vi "NI 9234 Calculations.vi"(9 "9234 Data in (V)":fxp<+/-,24,4>[](array[numeric])=[0.0, 0.0, 0.0, 0.0] format="%.22g", 10 "Acc mV/ms-2 Vals":sgl[](array[numeric])=[0.0, 0.0, 0.0, 0.0], 11 "Sample Length":u16) -> (0 "Freq":sgl[](array[numeric]), 1 "Peak":fxp<+/-,16,16>[](array[numeric]), 2 "RMS":fxp<+,16,16>[](array[numeric]), 3 "DC":fxp<+/-,16,16>[](array[numeric]))   [LabVIEW 2014]
uses:
  <vilib>/rvi/Analysis/common/FxpNativeNode/niFpgaFxpNative.xnode
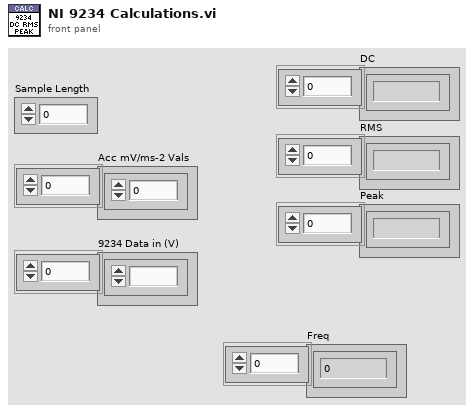
[diagram p1: front panel]
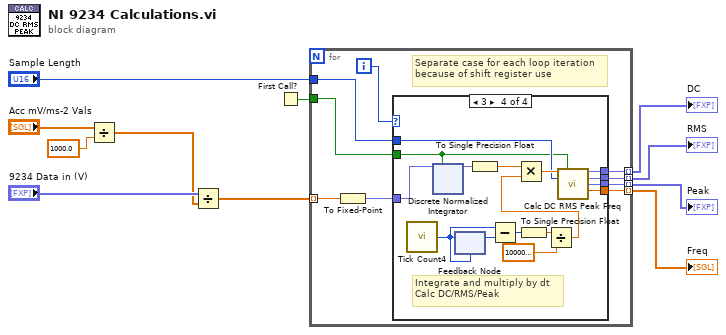
[diagram p0: block diagram]
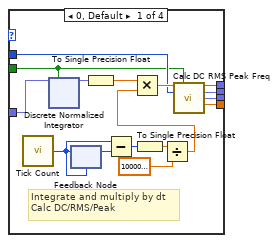
[diagram p2: hidden frame]
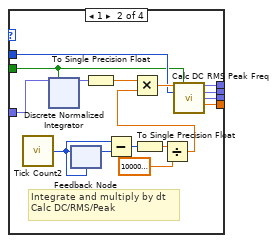
[diagram p3: hidden frame]
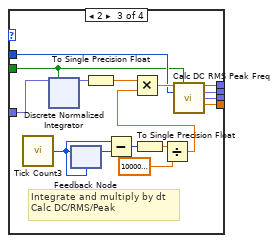
[diagram p4: hidden frame]
diagram:
  n1 = Divide(x="Acc mV/ms-2 Vals", y=sgl 1000.0 ("Numeric Control")) -> (x/y=w6:sgl[])
  n2 = Divide(x="9234 Data in (V)", y=w6) -> (x/y=w5:sgl[])
  n3 = First Call?() -> (First Call?: T/F=w10:bool)
  n4 = for {
    tunnel: w5 -> [w14] mode=indexing
    tunnel: w10 -> [w19]
    tunnel: [w18] -> w3 mode=indexing
    tunnel: [w17] -> w2 mode=indexing
    tunnel: [w16] -> w1 mode=indexing
    tunnel: "Sample Length" -> [w15]
    tunnel: [w12] -> w4 mode=indexing
    i -> [w20]
    # "Separate case for each loop iteration\nbecause of shift register use"
    n5 = To Fixed-Point(number=w14) -> (fixed-point=w13:fxp<+/-,32,16>)  [unwired: 1 in]
    n6 = case shown="3" w20 {
      tunnel: w13 -> [w36 w66 w96 w126]
      tunnel: w19 -> [w21 w51 w81 w111]
      tunnel: [w24 w54 w84 w114] -> w18
      tunnel: [w25 w55 w85 w115] -> w17
      tunnel: [w26 w56 w86 w116] -> w16
      tunnel: w15 -> [w22 w52 w82 w112]
      tunnel: [w27 w57 w87 w117] -> w12
      frame 0, Default {
        # "Integrate and multiply by dt\nCalc DC/RMS/Peak"
        n7 = call "Tick Count"() -> ("Tick Count(uSec)"=w33:u32)
        n8 = xnode ("Discrete Normalized Integrator")("input"=w36, "reset"=w21) -> ("output"=w35:fxp<+/-,48,32>)  [unwired: 1 in]
        n9 = feedback-in #1(w33) -> ()
        n10 = feedback #1(w33) -> (w34:u32)
        n11 = To Single Precision Float(number=w35) -> (single precision float=w29:sgl)
        n12 = Subtract(x=w33, y=w34) -> (x-y=w32:u32)
        n13 = To Single Precision Float(number=w32) -> (single precision float=w31:sgl)
        n14 = Divide(x=w31, y=sgl 1000000.0) -> (x/y=w28:sgl)
        n15 = Multiply(x=w29, y=w28) -> (x*y=w23:sgl)
        n16 = call "Calc DC RMS Peak Freq.vi"("input data"=w23, "reset"=w21, "Sample Size (1k)"=w22) -> ("DC"=w24:fxp<+/-,16,16>, "RMS"=w25:fxp<+,16,16>, "Peak"=w26:fxp<+/-,16,16>, "Frequency (Hz)"=w27:sgl)  [unwired: 8 in, 1 out]
      }
      frame 1 {
        # "Integrate and multiply by dt\nCalc DC/RMS/Peak"
        n17 = call "Tick Count2"() -> ("Tick Count(uSec)"=w63:u32)
        n18 = xnode ("Discrete Normalized Integrator")("input"=w66, "reset"=w51) -> ("output"=w65:fxp<+/-,48,32>)  [unwired: 1 in]
        n19 = feedback-in #2(w63) -> ()
        n20 = feedback #2(w63) -> (w64:u32)
        n21 = To Single Precision Float(number=w65) -> (single precision float=w59:sgl)
        n22 = Subtract(x=w63, y=w64) -> (x-y=w62:u32)
        n23 = To Single Precision Float(number=w62) -> (single precision float=w61:sgl)
        n24 = Divide(x=w61, y=sgl 1000000.0) -> (x/y=w58:sgl)
        n25 = Multiply(x=w59, y=w58) -> (x*y=w53:sgl)
        n26 = call "Calc DC RMS Peak Freq.vi"("input data"=w53, "reset"=w51, "Sample Size (1k)"=w52) -> ("DC"=w54:fxp<+/-,16,16>, "RMS"=w55:fxp<+,16,16>, "Peak"=w56:fxp<+/-,16,16>, "Frequency (Hz)"=w57:sgl)  [unwired: 8 in, 1 out]
      }
      frame 2 {
        # "Integrate and multiply by dt\nCalc DC/RMS/Peak"
        n27 = call "Tick Count3"() -> ("Tick Count(uSec)"=w93:u32)
        n28 = xnode ("Discrete Normalized Integrator")("input"=w96, "reset"=w81) -> ("output"=w95:fxp<+/-,48,32>)  [unwired: 1 in]
        n29 = feedback-in #3(w93) -> ()
        n30 = feedback #3(w93) -> (w94:u32)
        n31 = To Single Precision Float(number=w95) -> (single precision float=w89:sgl)
        n32 = Subtract(x=w93, y=w94) -> (x-y=w92:u32)
        n33 = To Single Precision Float(number=w92) -> (single precision float=w91:sgl)
        n34 = Divide(x=w91, y=sgl 1000000.0) -> (x/y=w88:sgl)
        n35 = Multiply(x=w89, y=w88) -> (x*y=w83:sgl)
        n36 = call "Calc DC RMS Peak Freq.vi"("input data"=w83, "reset"=w81, "Sample Size (1k)"=w82) -> ("DC"=w84:fxp<+/-,16,16>, "RMS"=w85:fxp<+,16,16>, "Peak"=w86:fxp<+/-,16,16>, "Frequency (Hz)"=w87:sgl)  [unwired: 8 in, 1 out]
      }
      frame 3 {
        # "Integrate and multiply by dt\nCalc DC/RMS/Peak"
        n37 = call "Tick Count4"() -> ("Tick Count(uSec)"=w123:u32)
        n38 = xnode ("Discrete Normalized Integrator")("input"=w126, "reset"=w111) -> ("output"=w125:fxp<+/-,48,32>)  [unwired: 1 in]
        n39 = feedback-in #4(w123) -> ()
        n40 = feedback #4(w123) -> (w124:u32)
        n41 = To Single Precision Float(number=w125) -> (single precision float=w119:sgl)
        n42 = Subtract(x=w123, y=w124) -> (x-y=w122:u32)
        n43 = To Single Precision Float(number=w122) -> (single precision float=w121:sgl)
        n44 = Divide(x=w121, y=sgl 1000000.0) -> (x/y=w118:sgl)
        n45 = Multiply(x=w119, y=w118) -> (x*y=w113:sgl)
        n46 = call "Calc DC RMS Peak Freq.vi"("input data"=w113, "reset"=w111, "Sample Size (1k)"=w112) -> ("DC"=w114:fxp<+/-,16,16>, "RMS"=w115:fxp<+,16,16>, "Peak"=w116:fxp<+/-,16,16>, "Frequency (Hz)"=w117:sgl)  [unwired: 8 in, 1 out]
      }
    }
  }
  "Freq" <- w4
  "DC" <- w3
  "RMS" <- w2
  "Peak" <- w1
